vi "PCO_GetDelayExposureTime.vi"(8 "error in (no error)":errorcluster {"code" format="%x"}, 11 "ph":u64) -> (0 "error out":errorcluster {"code" format="%x"}, 1 "dwDelay":u32, 2 "ErrorMessage":i32 format="%x", 3 "ph out":u64, 4 "wTimeBaseDelay":u16(ring) items=["ns", "us", "ms"], 5 "dwExposure":u32, 7 "wTimeBaseExposure":u16(ring) items=["ns", "us", "ms"])   [LabVIEW 2020, in "SDK.lvlib" / "TimingControl.lvlib"]
doc: "<b>Description:</b>\nThis function returns the current setting of the delay and exposure time values and the associated time base values.\nReturned values are only valid if last timing command was PCO_SetDelayExposureTime.\n\nDue to hardware limitations the returned values for the pco.edge, pco.1300 and pco.1400 are rounded values. To get exact timing values for the pco.edge please use function PCO_GetImageTiming.\n\n<b>Supported camera type:</b>\nAll cameras\n\n<b>Descriptor dependency:</b>\nNone"
uses:
  TimingControl.lvlib
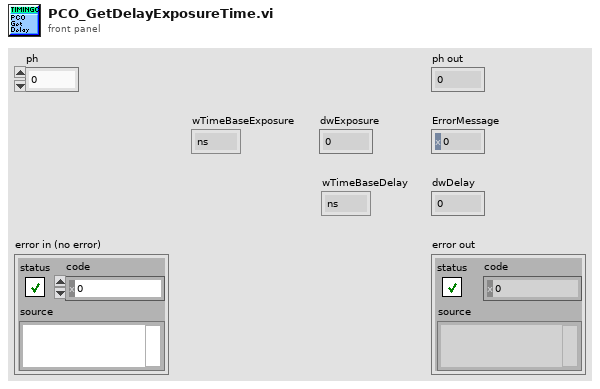
[diagram p1: front panel]
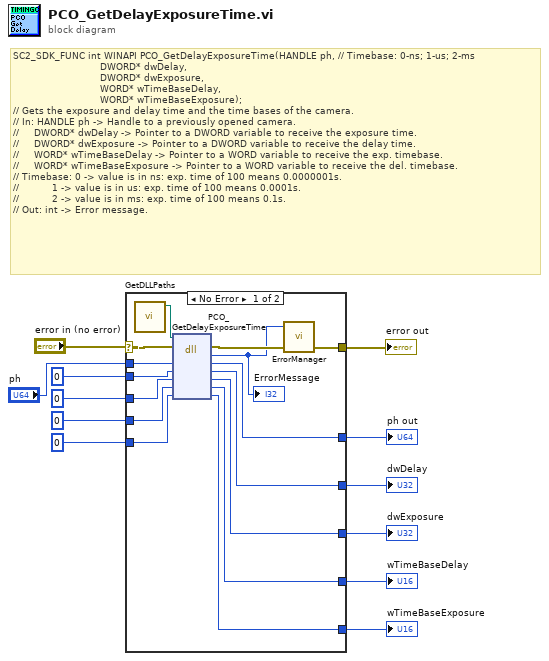
[diagram p0: block diagram]
diagram:
  # "SC2_SDK_FUNC int WINAPI PCO_GetDelayExposureTime(HANDLE ph, // Timebase: 0-ns; 1-us; 2-ms \n                             DWORD* dwDelay,\n                             DWORD* dwExposure,\n                             WORD* wTimeBaseDelay,\n                             WORD* wTimeBaseExposure);\n// Gets the exposure and delay time and the time bases of the camera.\n// In: HANDLE ph -> Handle to a previously opened camera.\n//     DWORD* dwDelay -> Pointer to a DWORD variable to receive the exposure time.\n//     DWORD* dwExposure -> Pointer to a DWORD variable to receive the delay time.\n//     WORD* wTimeBaseDelay -> Pointer to a WORD variable to receive the exp. timebase.\n//     WORD* wTimeBaseExposure -> Pointer to a WORD variable to receive the del. timebase.\n// Timebase: 0 -> value is in ns: exp. time of 100 means 0.0000001s.\n//           1 -> value is in us: exp. time of 100 means 0.0001s.\n//           2 -> value is in ms: exp. time of 100 means 0.1s.\n// Out: int -> Error message."
  n1 = case shown="No Error" "error in (no error)" {
    selector: "error in (no error)" -> [w17 w33]
    tunnel: "ph" -> [w27 w32]
    tunnel: [w26 w32] -> w11
    tunnel: u32 0 ("dwDelay") -> [w25 w31]
    tunnel: [w24 w31] -> w9
    tunnel: u32 0 ("dwExposure") -> [w23 w30]
    tunnel: [w22 w30] -> w7
    tunnel: u16 0 ("wTimeBaseDelay") -> [w21 w29]
    tunnel: [w20 w29] -> w5
    tunnel: u16 0 ("wTimeBaseExposure") -> [w19 w28]
    tunnel: [w18 w28] -> w3
    tunnel: [w15 w33] -> w2
    frame No Error {
      n2 = call "GetDLLPaths.vi"() -> ("SC2_Cam_Path"=w13:path)  [unwired: 9 in, 2 out]
      n3 = dll-call lib="?" fn="PCO_GetDelayExposureTime"(path in=w13, error in=w17, "ph"=w27, "dwDelay"=w25, "dwExposure"=w23, "wTimeBaseDelay"=w21, "wTimeBaseExposure"=w19) -> (error out=w16:errorcluster, "return type"=w14:i32, "ph"=w26:u64, "dwDelay"=w24:u32, "dwExposure"=w22:u32, "wTimeBaseDelay"=w20:u16, "wTimeBaseExposure"=w18:u16)  [unwired: 1 in, 1 out]
      "ErrorMessage" <- w14
      n4 = call "ErrorManager.vi"("error in (no error)"=w16, "error code"=w14) -> ("error out"=w15:errorcluster)  [unwired: 3 in]
    }
    frame Error {
    }
  }
  "ph out" <- w11
  "dwDelay" <- w9
  "dwExposure" <- w7
  "wTimeBaseDelay" <- w5
  "wTimeBaseExposure" <- w3
  "error out" <- w2
